vi "Write Voltage.vi"(8 "error in":errorcluster, 10 "Voltage":dbl, 11 "PowerSupply in":refnum<class "PowerSupply.lvclass">) -> (0 "error out":errorcluster, 3 "PowerSupply out":refnum<class "PowerSupply.lvclass">)   [LabVIEW 2019, in "PowerSupply.lvlib" / "PowerSupply.lvclass"]
uses:
  Library/PowerSupply.lvclass
  C:/Users/Public/Documents/Development/builds/Engine/Monitored Actor.lvlibp/Monitored Actor/Monitored Actor/Monitored Actor.lvclass
  Library/PowerSupply.lvclass/PowerSupply.ctl
  Read Settings.vi
  Private/Accessors/Read Limits.vi
  Write Settings.vi
  builds/Engine/Monitored Actor.lvlibp/Monitored Actor/Monitored Actor/Read Actor Label.vi
  builds/Instruments/Instruments.lvlibp/Library/Instruments.lvclass
  builds/Engine/Engine.lvlibp/Project/Engine.lvclass
  builds/Instruments/Instruments.lvlibp/Private/Polymorphic/Integers/Event from DBL.vi
  builds/Instruments/Instruments.lvlibp
  C:/Users/Public/Documents/Development/builds/Instruments/Instruments.lvlibp/Library/Instruments.lvclass
  C:/Users/Public/Documents/Development/builds/Tools/Config.lvlibp/Config.lvclass
  C:/Users/Public/Documents/Development/builds/Engine/Engine.lvlibp/Project/Engine.lvclass
  C:/Users/Public/Documents/Development/builds/Engine/Panel Manager.lvlibp/Panel Actor/Panel Actor.lvclass
  C:/Users/Public/Documents/Development/builds/Engine/Actor Framework.lvlibp/1abvi3w/vi.lib/ActorFramework/Actor/Actor.lvclass
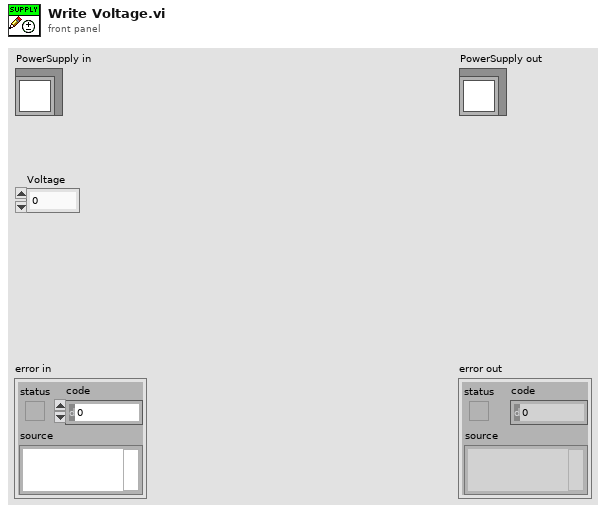
[diagram p1: front panel]
types:
  T1 = typedef "PowerSupply.lvlib/PowerSupply.lvclass/Settings.ctl" = cluster{"Voltage":dbl, "Current":dbl, "Output":bool, "OverVolt_Protect":dbl, "OverCurrent_Protect":dbl, "OVP":bool, "OCP":bool, "Interlock":bool, "Volt_Ramp":dbl, "Current_Ramp":dbl, "Sense Point":T2, "OCP Mode":T3}
  T2 = typedef "PowerSupply.lvlib/PowerSupply.lvclass/Sense Point.ctl" = enum16{"Local", "Remote"}
  T3 = typedef "PowerSupply.lvlib/PowerSupply.lvclass/OCP Mode.ctl" = enum16{"Shutdown", "Foldback"}
  T4 = typedef "PowerSupply.lvlib/PowerSupply.lvclass/Limits.ctl" = cluster{"Max_Current":dbl, "Max_Voltage":dbl, "Max_Current_Ramp":dbl, "Max_Voltage_Ramp":dbl, "Max_OCP":dbl, "Max_OVP":dbl}
  T5 = cluster{"Timestamp":timestamp, "Description":string, "Data":string}
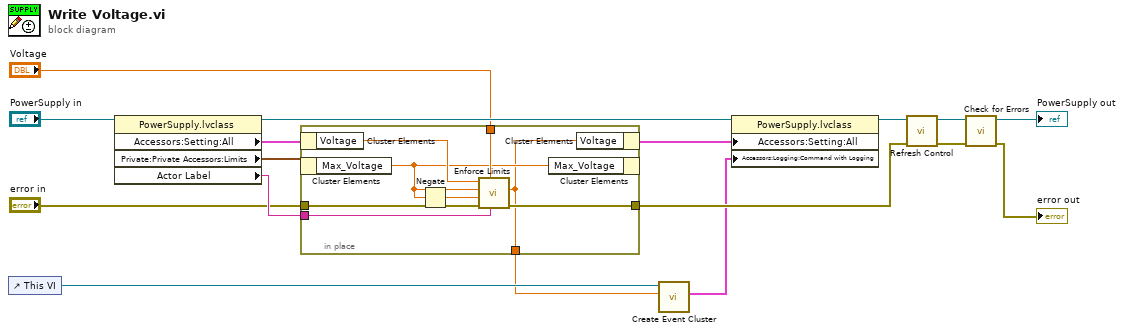
[diagram p0: block diagram]
diagram:
  n1 = control-ref of="This VI"() -> (w3:refnum<vi>)
  n2 = property class="PowerSupply.lvclass"(reference="PowerSupply in") -> (reference out=w17:refnum<class "PowerSupply.lvclass">, "Accessors:Setting:All"=w10:T1, "Private:Private Accessors:Limits"=w9:T4, "Actor Label"=w14:string)  [unwired: 1 in, 1 out]
  n3 = in-place {
    in-place-border: "Voltage" -> [w25]
    in-place-border: [w21] -> w11
    in-place-border: w14 -> [w20]
    in-place-border: "error in" -> [w19]
    in-place-border: [w18] -> w2
    n4 = in-place-cluster #1(w10) -> ("Voltage"=w24:dbl)
    n5 = in-place-cluster #2(w9) -> ("Max_Voltage"=w23:dbl)
    n6 = Negate(x=w23) -> (-x=w22:dbl)
    n7 = call "Enforce Limits.vi"("Device"=w20, "Setpoint"=w25, "error in"=w19, "Minimum"=w22, "Maximum"=w23, "Previous"=w24) -> ("error out"=w21:errorcluster, "Protected Setpoint"=w18:dbl)  [unwired: 4 in]
    n8 = in-place-cluster #2("Max_Voltage"=w23) -> ()  [unwired: 1 out]
    n9 = in-place-cluster #1("Voltage"=w18) -> (w16:T1)
  }
  n10 = call-poly "Create Event Cluster.vi"("Value"=w2, "VI Refnum"=w3) -> ("Event Data"=w1:T5)  [unwired: 9 in]
  n11 = property class="PowerSupply.lvclass"(reference=w17, "Accessors:Setting:All"=w16, "Accessors:Logging:Command with Logging"=w1) -> (reference out=w15:refnum<class "PowerSupply.lvclass">)  [unwired: 1 in, 1 out]
  n12 = call "Refresh Control.vi"("error in"=w11, "PowerSupply in"=w15) -> ("error out"=w13:errorcluster, "PowerSupply out"=w12:refnum<class "PowerSupply.lvclass">)  [unwired: 8 in]
  n13 = call "Check for Errors.vi"("error in"=w13, "Engine in"=w12) -> ("error out"=→"error out":errorcluster, "Engine out"=→"PowerSupply out":refnum<class "PowerSupply.lvclass">)  [unwired: 8 in]
